vi "Land Cmd Detect (SubVI).vi"(1 "Read String":string) -> (0 "Land Command":bool)   [LabVIEW 2014]
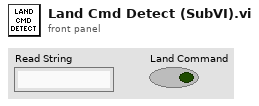
[diagram p1: front panel]
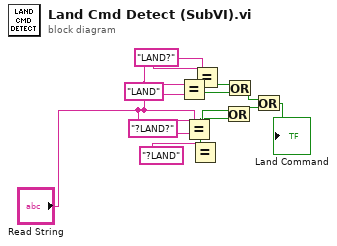
[diagram p0: block diagram]
diagram:
  n1 = Equal?(x="Read String", y="LAND") -> (x = y?=w9:bool)
  n2 = Equal?(x="Read String", y="?LAND?") -> (x = y?=w7:bool)
  n3 = Equal?(x="Read String", y="?LAND") -> (x = y?=w6:bool)
  n4 = Equal?(x="Read String", y="LAND?") -> (x = y?=w8:bool)
  n5 = Or(x=w7, y=w6) -> (x .or. y?=w10:bool)
  n6 = Or(x=w8, y=w9) -> (x .or. y?=w11:bool)
  n7 = Or(x=w11, y=w10) -> (x .or. y?=→"Land Command":bool)
